vi "Detector Get Image.vi"(8 "error in (no error)":errorcluster, 11 "RIMAS Detector in":refnum<class "RIMAS Detector.lvclass">) -> (0 "error out":errorcluster, 1 "FITS Detector Settings":T2, 2 "Images":T3[](array[typedef]) {"Detector #" items=["None", "YJ", "HK"]}, 3 "RIMAS Detector out":refnum<class "RIMAS Detector.lvclass">, 4 "Message Log":string, 6 "Detector Files":T1)   [LabVIEW 2022 SP3, in "RIMAS Detector.lvclass"]
uses:
  RIMAS Detector.lvclass
  C:/Development/rimas/RIMAS/Detector/Detector Class/Detector Class.lvclass
  Detector Image typedef cluster.ctl
  RIMAS Observation Config.ctl
  Detector cluster Files.ctl
  Detector Class.lvclass
  RIMAS Detector.lvclass/RIMAS Detector.ctl
panel:
  out "data out 2":string
  out "data out":string
  # "sec"
  # "sec"
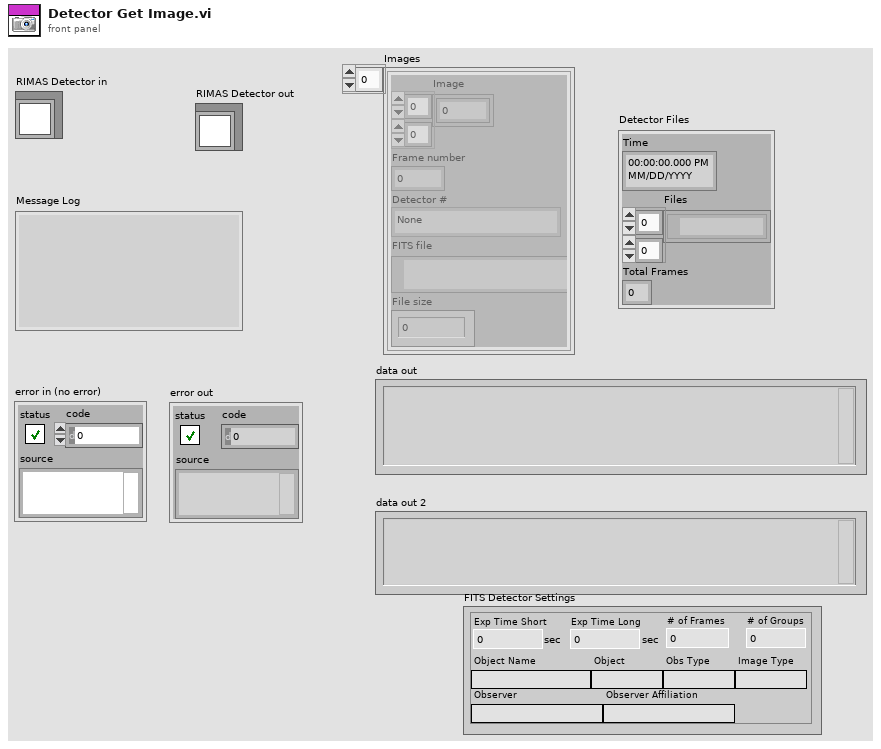
[diagram p1: front panel]
types:
  T1 = typedef "Detector Class.lvclass/Detector cluster Files.ctl" = cluster{"Time":timestamp, "Files":path[][], "Total Frames":i32}
  T2 = typedef "RIMAS Observation Config.ctl" = cluster{"Exp Time Short":dbl, "# of Frames":dbl, "Exp Time Long":dbl, "# of Groups":dbl, "Object Name":string, "Object":string, "Obs Type":string, "Image Type":string, "Observer":string, "Observer Affiliation":string}
  T3 = typedef "Detector Class.lvclass/Detector Image typedef cluster.ctl" = cluster{"Image":sgl[][], "Frame number":i32, "Detector #":u16, "FITS file":path, "File size":i64}
  T4 = typedef "RIMAS Detector Config.ctl" = cluster{"Detector":u16, "Offsets":u16[][], "Detector Computer":T5, "FITS hdr template0":path, "FITS hdr template1":path, "FITS Data File Path":path, "FITS Detector Settings":T2, "Sim Folder":path, "Integration Mode":T6, "Integration Time":dbl, "Frame Int Time":dbl}
  T5 = typedef "RIMAS Detector Server Config.ctl" = cluster{"Machine":string, "Password":string, "FITS File Path":string, "Port":u16, "Header Path":string, "Name":string}
  T6 = typedef "Detector enum Detector Integration Mode.ctl" = enum16{"SSR", "CDS", "MEAN", "MEDIAN", "MODE", "MIIN", "MAX"}
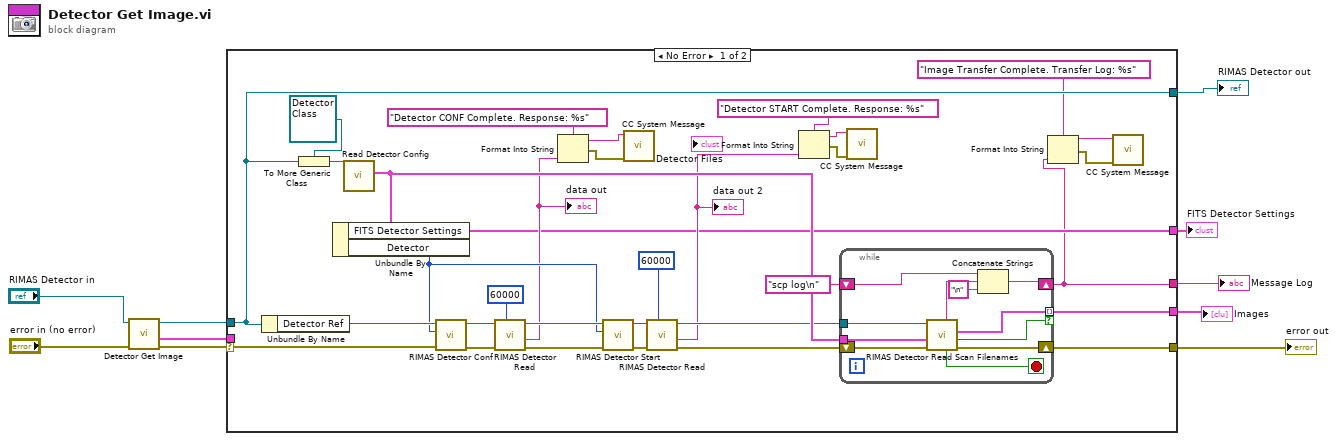
[diagram p0: block diagram]
diagram:
  n1 = call-parent "Detector Get Image.vi"("error in (no error)"="error in (no error)", "Detector Class in"="RIMAS Detector in") -> ("error out"=w8:errorcluster, "FITS Detector Settings"=w3:T2, "Detector Class out"=w7:refnum<class "RIMAS Detector.lvclass">)  [unwired: 4 in, 3 out]
  n2 = case shown="No Error" w8 {
    selector: w8 -> [w24 w56]
    tunnel: w7 -> [w41 w57]
    tunnel: [w41 w57] -> w6
    tunnel: [w11 _] -> w4
    tunnel: [w40 w56] -> w5
    tunnel: w3 -> [_ w55]
    tunnel: [w33 _] -> w2
    tunnel: [w12 w55] -> w1
    frame No Error {
      n3 = Unbundle By Name(w41) -> ("Detector Ref"=w32:refnum<k5>)
      n4 = To More Generic Class(target class=refnum<class "Detector Class.lvclass"> refnum ("Detector Class.lvclass"), reference=w41) -> (generic class reference=w42:refnum<class "Detector Class.lvclass">)
      n5 = call-dynamic "Read Detector Config.vi"("Detector Class in"=w42) -> ("Detector Config"=w39:T4)  [unwired: 8 in, 2 out]
      n6 = Unbundle By Name(w39) -> ("FITS Detector Settings"=w12:T2, "Detector"=w25:u16)
      n7 = call "RIMAS Detector Conf.vi"("Error In"=w24, "Detector"=w25, "Detector Ref in"=w32) -> ("Error Out"=w31:errorcluster, "Detector Ref out"=w30:refnum<k5>)  [unwired: 7 in]
      n8 = call "RIMAS Detector Read.vi"("timeout (ms)"=60000, "Error In"=w31, "Detector Ref"=w30) -> ("Error Out"=w29:errorcluster, "First String"=w22:string, "Detector Ref dup"=w28:refnum<k5>)  [unwired: 5 in, 1 out]
      "data out" <- w22
      n9 = Format Into String(format string="Detector CONF Complete. Response: %s", w22) -> (resulting string=w21:string, error out=w16:errorcluster)  [unwired: 2 in]
      n10 = call "RIMAS Detector Start.vi"("Error In"=w29, "Detector"=w25, "Detector Ref in"=w28) -> ("Error Out"=w26:errorcluster, "Detector Ref out"=w27:refnum<k5>)  [unwired: 7 in]
      n11 = call "CC System Message.vi"("error in (no error)"=w16, "Message"=w21) -> ()  [unwired: 9 in, 1 out]
      n12 = call "RIMAS Detector Read.vi"("timeout (ms)"=60000, "Error In"=w26, "Detector Ref"=w27) -> ("Error Out"=w37:errorcluster, "First String"=w19:string, "Detector Ref dup"=w38:refnum<k5>)  [unwired: 5 in, 1 out]
      "data out 2" <- w19
      n13 = Format Into String(format string="Detector START Complete. Response: %s", w19) -> (resulting string=w17:string, error out=w18:errorcluster)  [unwired: 2 in]
      n14 = while {
        tunnel: w39 -> [w53]
        tunnel: w38 -> [w52]
        shift-right: [w54] -> w40
        shift-left: w37 -> [w51]
        tunnel: [w50] -> w33 mode=indexing if=w44
        shift-right: [w46] -> w11
        shift-left: "scp log\n" -> [w48]
        stop <- w45 stop-if-true
        n15 = call "RIMAS Detector Read Scan Filenames.vi"("Error In"=w51, "Detector Config"=w53, "Detector Ref"=w52) -> ("Error Out"=w54:errorcluster, "Image OK"=w44:bool, "Image Data"=w50:T3, "Done"=w45:bool, "Log"=w49:string)  [unwired: 3 in, 1 out]
        n16 = Concatenate Strings(w48, w49, "\n" ("string")) -> (w46:string)
      }
      n17 = call "CC System Message.vi"("error in (no error)"=w18, "Message"=w17) -> ()  [unwired: 9 in, 1 out]
      n18 = Format Into String(format string="Image Transfer Complete. Transfer Log: %s", w11) -> (resulting string=w14:string, error out=w15:errorcluster)  [unwired: 2 in]
      n19 = call "CC System Message.vi"("error in (no error)"=w15, "Message"=w14) -> ()  [unwired: 9 in, 1 out]
    }
    frame Error {
    }
  }
  "error out" <- w5
  "RIMAS Detector out" <- w6
  "Images" <- w2
  "Message Log" <- w4
  "FITS Detector Settings" <- w1
